vi "Read Delimited Spreadsheet (DBL).vi"(0 "file path (dialog if empty)":path, 1 "format (%.3f)":string="%.3f", 5 "number of rows (all:-1)":i32=-1, 7 "start of read offset (chars.:0)":i32, 9 "max characters/row  (no limit:0)":i32, 11 "error in (no error)":errorcluster, 12 "transpose? (F)":bool, 13 "delimiter (\\t)":string="\t") -> (4 "new file path (Not A Path if cancelled)":path, 6 "all rows":dbl[][](array[numeric]), 8 "first row":dbl[](array[numeric]), 10 "mark after read (chars.)":i32, 14 "EOF?":bool, 15 "error out":errorcluster)   [LabVIEW 2020]
doc: "Reads a specified number of lines or rows from a numeric text file beginning at a specified character offset and converts the data to a 2D, double-precision array of numbers, strings, or integers. You must manually select the polymorphic instance you want to use."
panel:
  in  "type (empty)":dbl[][](array[numeric]) format="%0.2f"
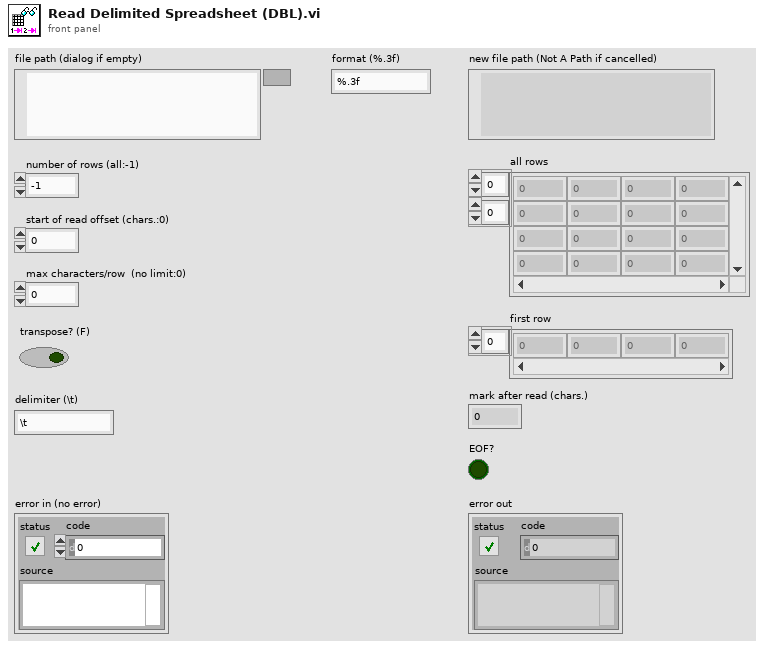
[diagram p1: front panel]
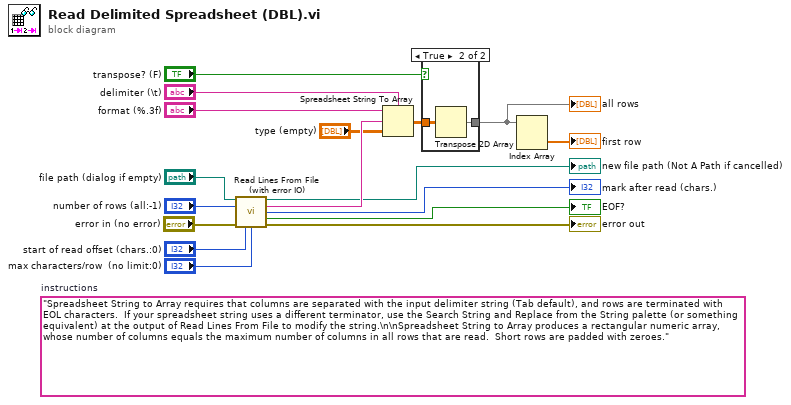
[diagram p0: block diagram]
diagram:
  (unwired) "Spreadsheet String to Array requires that columns are separated with the input delimiter string (Tab default), and rows are terminated with EOL characters.  If your spreadsheet string uses a different terminator, use the Search String and Replace from the String palette (or something equivalent) at the output of Read Lines From File to modify the string.\n\nSpreadsheet String to Array produces a rectangular numeric array, whose number of columns equals the maximum number of columns in all rows that are read.  Short rows are padded with zeroes."  # instructions
  n1 = call "Read Lines From File (with error IO).vi"("file path (dialog if empty)"="file path (dialog if empty)", "number of rows (all:-1)"="number of rows (all:-1)", "error in (no error)"="error in (no error)", "start of read offset (chars.:0)"="start of read offset (chars.:0)", "max characters/row  (no limit:0)"="max characters/row  (no limit:0)") -> ("new file path (Not A Path if cancelled)"=→"new file path (Not A Path if cancelled)":path, "line string"=w13:string, "mark after read (chars.)"=→"mark after read (chars.)":i32, "EOF?"=→"EOF?":bool, "error out"=→"error out":errorcluster)  [unwired: 6 in]
  n2 = Spreadsheet String To Array(delimiter (Tab)="delimiter (\\t)", format string="format (%.3f)", spreadsheet string=w13, array type (2D Dbl)="type (empty)") -> (array=w11:dbl[][])
  n3 = case shown="True" "transpose? (F)" {
    tunnel: [w18 w20] -> w9
    tunnel: w11 -> [w18 w19]
    frame False {
    }
    frame True {
      n4 = Transpose 2D Array(2D array=w19) -> (transposed array=w20:dbl[][])
    }
  }
  "all rows" <- w9
  n5 = Index Array(array=w9) -> (element=→"first row":dbl[])  [unwired: 2 in]
